vi "Verify Host Buffers Size.vi"(4 "output.Host Buffer Size":u32, 6 "input.Host Buffer Size":u32, 8 "error in":errorcluster) -> (0 "error out":errorcluster)   [LabVIEW 2013]
doc: "This VI verifies that the Host Buffer Depths for both the Input FIFO and Output FIFO are the same."
uses:
  <vilib>/ErrorRing/Error Ring.xnode
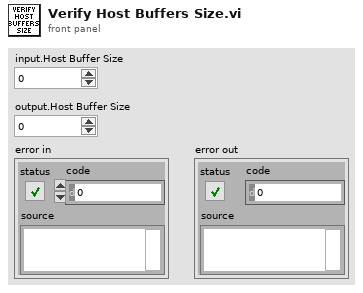
[diagram p1: front panel]
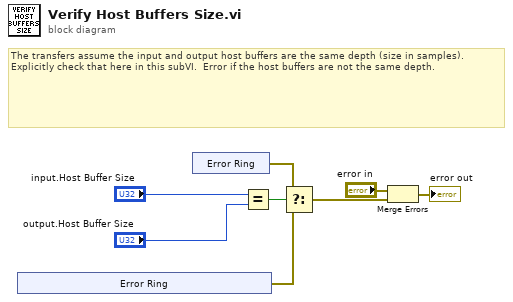
[diagram p0: block diagram]
diagram:
  # "The transfers assume the input and output host buffers are the same depth (size in samples).  Explicitly check that here in this subVI.  Error if the host buffers are not the same depth."
  n1 = xnode "Error Ring"() -> ("error out"=w3:errorcluster)
  n2 = xnode "Error Ring"() -> ("error out"=w7:errorcluster)
  n3 = Equal?(x="input.Host Buffer Size", y="output.Host Buffer Size") -> (x = y?=w8:bool)
  n4 = Select(t=w7, s=w8, f=w3) -> (s? t:f=w4:errorcluster)
  n5 = Merge Errors("error in", w4) -> (→"error out":errorcluster)
